vi "Client 3.vi"() -> ()   [LabVIEW 2019, in "RemoteControl.ZMQ.lvclass"]
uses:
  RemoteControl.ZMQ.lvclass
panel:
  in  "milliseconds to wait":u32
  out "Command Sent":string
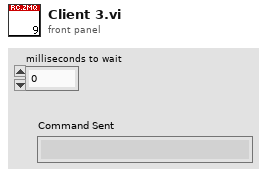
[diagram p1: front panel]
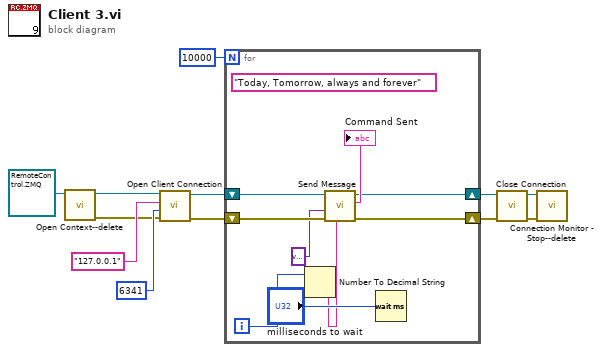
[diagram p0: block diagram]
diagram:
  n1 = call-dynamic "Open Context--delete.vi"("RemoteControl.ZMQ in"=refnum<class "RemoteControl.ZMQ.lvclass"> refnum) -> ("error out"=w1:errorcluster, "RemoteControl.ZMQ out"=w2:refnum<class "RemoteControl.ZMQ.lvclass">)  [unwired: 9 in]
  n2 = call-dynamic "Open Client Connection.vi"("error in (no error)"=w1, "Port"=u16 6341, "address"="127.0.0.1" ("Address"), "RemoteControl.ZMQ in"=w2) -> ("error out"=w10:errorcluster, "RemoteControl.ZMQ out"=w11:refnum<class "RemoteControl.ZMQ.lvclass">)  [unwired: 6 in]
  n3 = for {
    N: 10000 -> [_]
    shift-right: [w17] -> w7
    shift-left: w11 -> [w21]
    shift-right: [w16] -> w6
    shift-left: w10 -> [w20]
    i -> [w15]
    (unwired) "Today, Tomorrow, always and forever" ("Command")
    n4 = Number To Decimal String(number=w15) -> (decimal integer string=w13:string)  [unwired: 1 in]
    n5 = call-dynamic "Send Message.vi"("ID"=w13, "error in (no error)"=w20, "Data"=variant, "RemoteControl.ZMQ in"=w21) -> ("error out"=w16:errorcluster, "ACK"=→"Command Sent":string, "RemoteControl.ZMQ out"=w17:refnum<class "RemoteControl.ZMQ.lvclass">)  [unwired: 5 in]
    n6 = Wait (ms)(milliseconds to wait="milliseconds to wait") -> ()  [unwired: 1 out]
  }
  n7 = call-dynamic "Close Connection.vi"("error in (no error)"=w6, "RemoteControl.ZMQ in"=w7) -> ("error out"=w8:errorcluster, "RemoteControl.ZMQ out"=w9:refnum<class "RemoteControl.ZMQ.lvclass">)  [unwired: 8 in]
  n8 = call-dynamic "Connection Monitor - Stop--delete.vi"("error in (no error)"=w8, "RemoteControl.ZMQ in"=w9) -> ()  [unwired: 8 in, 2 out]
